vi "Autonomous.vi"   [LabVIEW 2018]
doc: "This VI starts when autonomous period begins, and will automatically be terminated when it ends. You can carry out timed or sensor driven operations directly to I/O or to subsystems without needing to return to the caller."
uses:
  <vilib>/Rock Robotics/WPI/DriverStation/WPI_DriverStationDerivedRobotMode.ctl
  Dashboard-Project/CustomThings/Routine.ctl
  <vilib>/Rock Robotics/WPI/Utilities/WPI_GetSetVariantRefNum.vi
  Framework/Robot Global Data.vi
  <vilib>/Rock Robotics/Network Tables/NT Read Number.vi
types:
  T1 = typedef "Routine.ctl" = enum16{"Do Left Rocket", "Do Right Rocket", "Do Left Cargo Ship Panels", "Do Right Cargo Ship Panels", "Do Front Left Cargo Ship", "Do Front Right Cargo Ship", "Do Teleop"}
  T2 = typedef "Command Status Info.ctl" = cluster{"Name":string, "Status":T3, "notifier out":T4}
  T3 = typedef "Completion Status.ctl" = enum16{"Successful", "Aborted", "Incomplete"}
  T4 = typedef "Completion Notifier.ctl" = refnum<notifier>
  T5 = typedef "WPI_JoystickDevRef.ctl" = cluster{"Device":T6}
  T6 = typedef "WPI_JoystickDeviceEnum.ctl" = enum16{"USB 0", "USB 1", "USB 2", "USB 3", "USB 4", "USB 5"}
  T7 = typedef "WPI_DriverStationDerivedRobotMode.ctl" = enum16{"Init", "Execute", "Stop"}
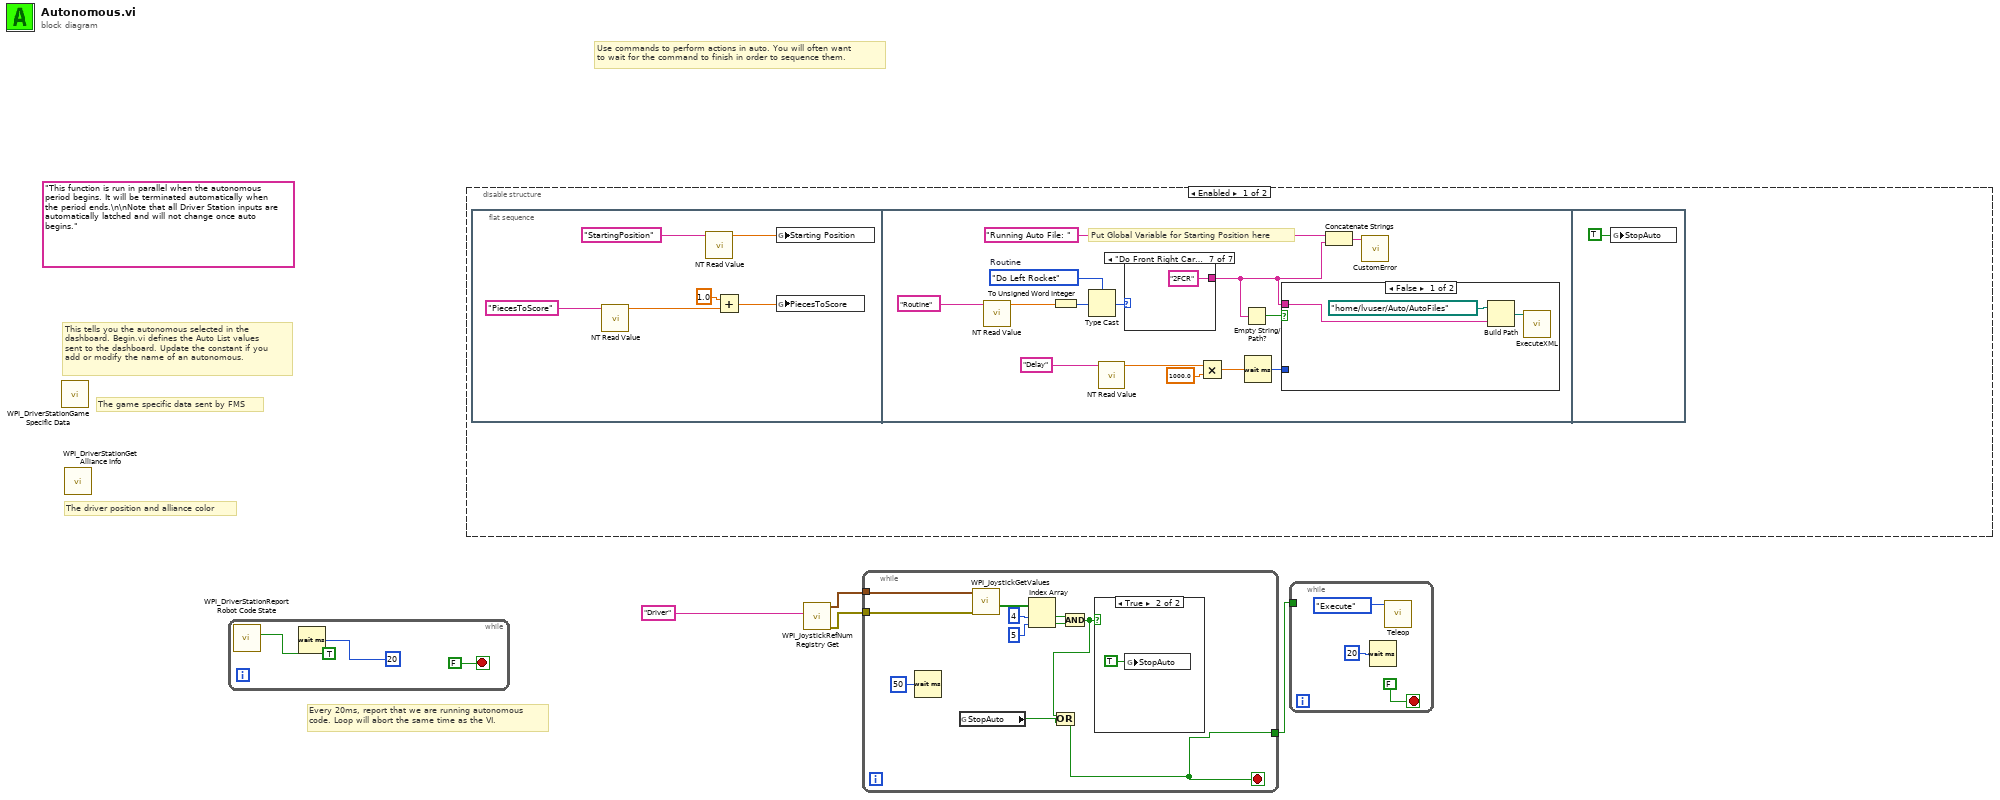
[diagram p0: block diagram]
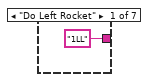
[diagram p3: hidden frame]
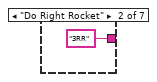
[diagram p4: hidden frame]
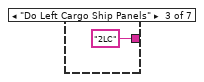
[diagram p5: hidden frame]
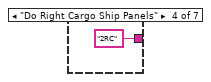
[diagram p6: hidden frame]
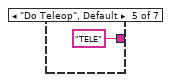
[diagram p7: hidden frame]
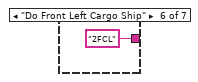
[diagram p8: hidden frame]
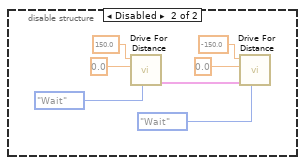
[diagram p9: hidden frame]
diagram:
  (unwired) "This function is run in parallel when the autonomous period begins. It will be terminated automatically when the period ends.\n\nNote that all Driver Station inputs are automatically latched and will not change once auto begins."
  # "The game specific data sent by FMS"
  # "This tells you the autonomous selected in the \ndashboard. Begin.vi defines the Auto List values\nsent to the dashboard. Update the constant if you\nadd or modify the name of an autonomous."
  # "Every 20ms, report that we are running autonomous\ncode. Loop will abort the same time as the VI."
  # "Use commands to perform actions in auto. You will often want\nto wait for the command to finish in order to sequence them."
  # "The driver position and alliance color"
  n1 = call <vilib>:"WPI_DriverStationGame Specific Data.vi"() -> ()  [unwired: 11 in, 1 out]
  n2 = call <vilib>:"WPI_DriverStationGet Alliance Info.vi"() -> ()  [unwired: 12 out]
  n3 = while {
    stop <- FALSE stop-if-true
    n4 = call <vilib>:"WPI_DriverStationReport Robot Code State.vi"("Autonomous"=TRUE) -> ()  [unwired: 10 in, 1 out]
    n5 = Wait (ms)(milliseconds to wait=u32 20) -> ()  [unwired: 1 out]
  }
  n6 = disable-structure shown="Enabled" {
    frame Enabled {
      n7 = flat-sequence {
        frame #0 {
          n8 = call-poly <vilib>:"NT Read Value.vi"("Name"="PiecesToScore") -> ("Numeric"=w9:dbl)  [unwired: 9 in, 1 out]
          n9 = call-poly <vilib>:"NT Read Value.vi"("Name"="StartingPosition") -> ("Numeric"=w8:dbl)  [unwired: 9 in, 1 out]
          n10 = Add(x=1.0, y=w9) -> (x+y=w12:dbl)
          n11 = global write "Robot Global Data.vi" "Starting Position"(w8) -> ()
          n12 = global write "Robot Global Data.vi" "PiecesToScore"(w12) -> ()
        }
        frame #1 {
          w24 = Routine."Do Left Rocket"  # Routine
          # "Put Global Variable for Starting Position here"
          n13 = call-poly <vilib>:"NT Read Value.vi"("Name"="Routine") -> ("Numeric"=w26:dbl)  [unwired: 9 in, 1 out]
          n14 = To Unsigned Word Integer(number=w26) -> (unsigned 16bit integer=w25:u16)
          n15 = Type Cast(type=w24, x=w25) -> (*(type *) &x=w23:T1)
          n16 = call-poly <vilib>:"NT Read Value.vi"("Name"="Delay") -> ("Numeric"=w19:dbl)  [unwired: 9 in, 1 out]
          n17 = case shown="\"Do Front Right Cargo Ship\"" w23 {
            tunnel: ["1LL" ("name or relative path") "3RR" ("name or relative path") "2LC" ("name or relative path") "2RC" ("name or relative path") "TELE" ("name or relative path") "2FCL" ("name or relative path") "2FCR" ("name or relative path")] -> w16
            frame "Do Left Rocket" {
            }
            frame "Do Right Rocket" {
            }
            frame "Do Left Cargo Ship Panels" {
            }
            frame "Do Right Cargo Ship Panels" {
            }
            frame "Do Teleop", Default {
            }
            frame "Do Front Left Cargo Ship" {
            }
            frame "Do Front Right Cargo Ship" {
            }
          }
          n18 = Multiply(x=w19, y=1000.0) -> (x*y=w18:dbl)
          n19 = Empty String/Path?(string/path=w16) -> (empty?=w22:bool)
          n20 = Wait (ms)(milliseconds to wait=w18) -> (millisecond timer value=w17:u32)
          n21 = case shown="False" w22 {
            tunnel: w16 -> [w28 _]
            tunnel: w17 -> [_ _]
            frame False {
              n22 = Build Path(base path=path "/home/lvuser/Auto/AutoFiles", name or relative path=w28) -> (appended path=w30:path)
              n23 = call "ExecuteXML.vi"("Auto File Path"=w30) -> ()  [unwired: 10 in, 1 out]
            }
            frame True {
            }
          }
          n24 = Concatenate Strings("Running Auto File: " ("string"), w16) -> (w15:string)
          n25 = call "CustomError.vi"("String"=w15) -> ()  [unwired: 10 in, 1 out]
        }
        frame #2 {
          n26 = global write "Robot Global Data.vi" "StopAuto"(TRUE) -> ()
        }
      }
    }
    frame Disabled {
      n27 = call "Drive For Distance.vi"("Synchronication"=enum16{"Start", "Wait"}."Wait", "Angle"=0.0, "Distance"=150.0) -> ("Command Info Out"=w39:T2)  [unwired: 8 in]
      n28 = call "Drive For Distance.vi"("Synchronication"=enum16{"Start", "Wait"}."Wait", "Command Info In"=w39, "Angle"=0.0, "Distance"=-150.0) -> ()  [unwired: 7 in, 1 out]
    }
  }
  n29 = call <vilib>:"WPI_JoystickRefNum Registry Get.vi"("refnum name"="Driver") -> ("error out"=w3:errorcluster, "JoystickDevRef"=w4:T5)  [unwired: 9 in]
  n30 = while {
    tunnel: w3 -> [w51]
    tunnel: w4 -> [w50]
    tunnel: [w46] -> w1
    stop <- w46 stop-if-true
    n31 = Wait (ms)(milliseconds to wait=u32 50) -> ()  [unwired: 1 out]
    n32 = global read "Robot Global Data.vi" "StopAuto"() -> (w48:bool)
    n33 = call <vilib>:"WPI_JoystickGetValues.vi"("error in (no error)"=w51, "JoystickDevRef"=w50) -> ("Buttons"=w54:bool[])  [unwired: 5 in, 4 out]
    n34 = Index Array(array=w54, index #1=4 ("index"), index #2=5 ("index")) -> (element #1=w55:bool, element #2=w56:bool)
    n35 = And(x=w55, y=w56) -> (x .and. y?=w47:bool)
    n36 = Or(x=w47, y=w48) -> (x .or. y?=w46:bool)
    n37 = case shown="True" w47 {
      frame False {
      }
      frame True {
        n38 = global write "Robot Global Data.vi" "StopAuto"(TRUE ("StopAuto")) -> ()
      }
    }
  }
  n39 = while {
    tunnel: w1 -> [_]
    stop <- FALSE stop-if-true
    n40 = Wait (ms)(milliseconds to wait=u32 20) -> ()  [unwired: 1 out]
    n41 = call "Teleop.vi"("Call Context"=WPI_DriverStationDerivedRobotMode."Execute") -> ()  [unwired: 11 in]
  }
